vi "destroy.vi"(8 "error in (no error)":errorcluster, 11 "Laser View in":refnum<class "Laser View.lvclass">) -> (0 "error out":errorcluster, 3 "Laser View out":refnum<class "Laser View.lvclass">)   [LabVIEW 2022 SP3, in "Laser View.lvclass"]
uses:
  Laser View.lvclass
  Laser View.lvclass/Laser View.ctl
  iView/base view/base view.lvclass
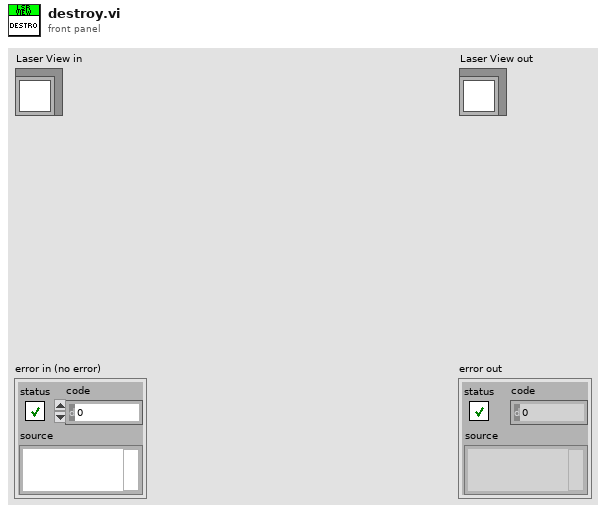
[diagram p1: front panel]
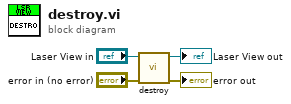
[diagram p0: block diagram]
diagram:
  n1 = call-parent "destroy.vi"("error in (no error)"="error in (no error)", "base view in"="Laser View in") -> ("error out"=→"error out":errorcluster, "base view out"=→"Laser View out":refnum<class "Laser View.lvclass">)  [unwired: 8 in]
